vi "Launch Async.vi"(8 "error in (no error)":errorcluster, 10 "Device Ref in":T8 format="%.0x", 11 "RT Data in":T1 {"Channels"."Voltage"."Ref"."Data Reference" format="%.0x"; "Channels"."Current"."Ref"."Data Reference" format="%.0x"; "Channels"."Read Volt"."Ref" format="%.0x"; "Channels"."Mode"."Ref" format="%.0x"}) -> (0 "error out":errorcluster, 2 "Device Ref out":T8 format="%.0x", 3 "RT Data out":T1 {"Channels"."Voltage"."Ref"."Data Reference" format="%.0x"; "Channels"."Current"."Ref"."Data Reference" format="%.0x"; "Channels"."Read Volt"."Ref" format="%.0x"; "Channels"."Mode"."Ref" format="%.0x"})   [LabVIEW 2011, in "Switch-DMM Custom Device.lvlib"]
uses:
  Switch-DMM Custom Device.lvlib
  <vilib>/NI Veristand/Custom Device API/Custom Device Item Ref.ctl
  Controls/RT Data.ctl
  Controls/Channels.ctl
  Controls/Single Channel.ctl
  <vilib>/NI Veristand/Custom Device API/Data Reference.ctl
  Controls/Block Channels.ctl
  <vilib>/NI Veristand/Custom Device API/Block Data Reference.ctl
  Controls/Communication.ctl
  Controls/Async Status.ctl
  Controls/Async State.ctl
  Controls/Async Command.ctl
  Controls/Async Events.ctl
  Controls/Async Data.ctl
  Controls/Hardware.ctl
  <instrlib>/niDMM/nidmm.llb/niDMM Resolution in Digits.ctl
  <vilib>/NI Veristand/Custom Device API/Custom Device API.lvlib
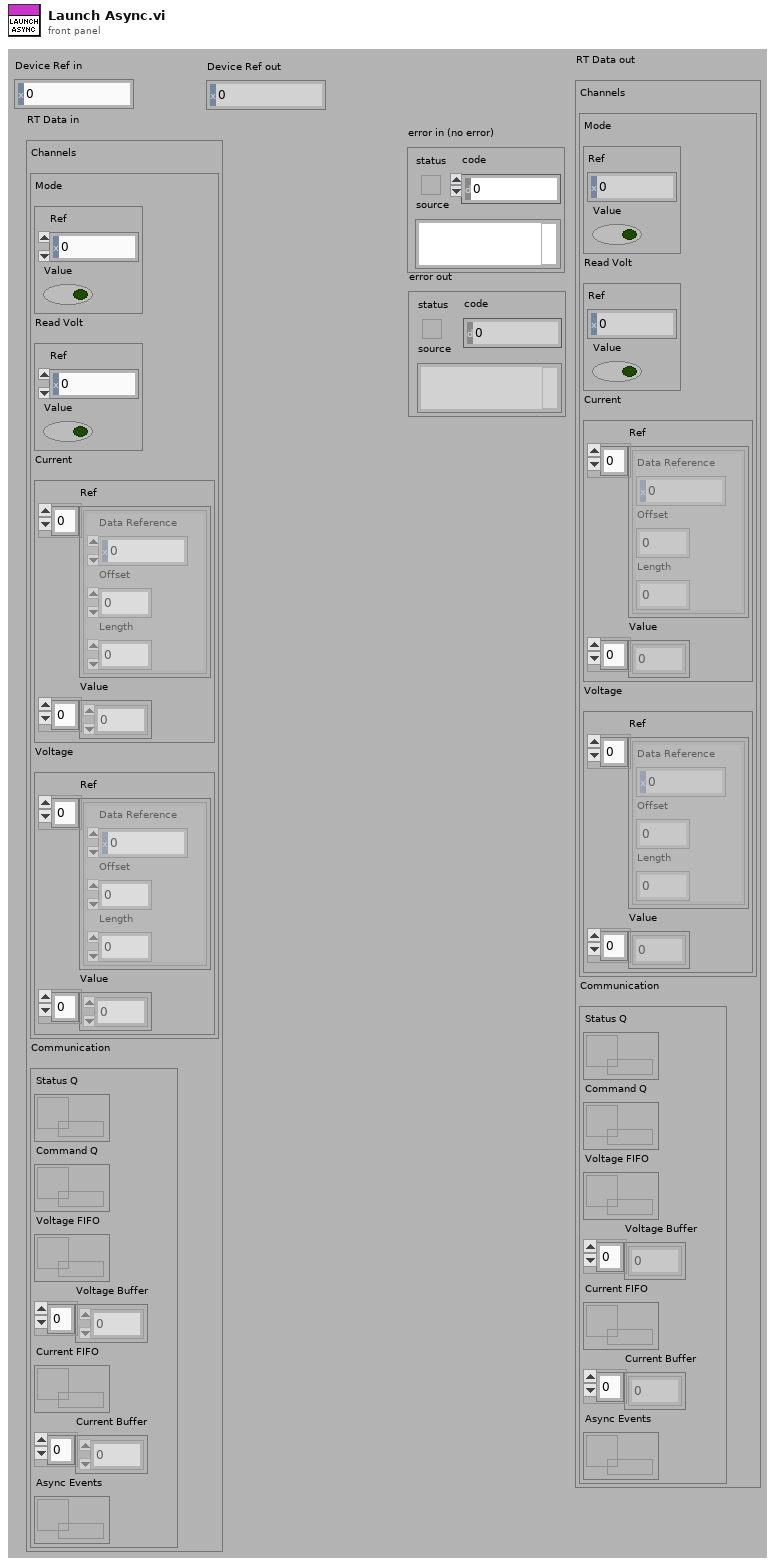
[diagram p1: front panel]
types:
  T1 = typedef "Switch-DMM Custom Device.lvlib/RT Data.ctl" = cluster{"Channels":T2, "Communication":T7}
  T2 = typedef "Switch-DMM Custom Device.lvlib/Channels.ctl" = cluster{"Mode":T3, "Read Volt":T3, "Current":T5, "Voltage":T5}
  T3 = typedef "Switch-DMM Custom Device.lvlib/Single Channel.ctl" = cluster{"Ref":T4, "Value":bool}
  T4 = typedef "Custom Device API.lvlib/Data Reference.ctl" = i32
  T5 = typedef "Switch-DMM Custom Device.lvlib/Block Channels.ctl" = cluster{"Ref":T6[], "Value":dbl[]}
  T6 = typedef "Custom Device API.lvlib/Block Data Reference.ctl" = cluster{"Data Reference":T4, "Offset":i32, "Length":i32}
  T7 = typedef "Switch-DMM Custom Device.lvlib/Communication.ctl" = cluster{"Status Q":refnum<queue>, "Command Q":refnum<queue>, "Voltage FIFO":refnum<k33>, "Voltage Buffer":dbl[], "Current FIFO":refnum<k33>, "Current Buffer":dbl[], "Async Events":refnum<queue>}
  T8 = typedef "Custom Device API.lvlib/Custom Device Item Ref.ctl" = u64
  T9 = typedef "Switch-DMM Custom Device.lvlib/Async Data.ctl" = cluster{"Hardware":T10, "Communication":T7}
  T10 = typedef "Switch-DMM Custom Device.lvlib/Hardware.ctl" = cluster{"Switch Device":refnum<k15>, "DMM Device":refnum<k15>, "DMM -> Switch Trigger":u16, "Switch -> DMM Trigger":u16, "Sample Interval (sec)":dbl, "Current Samples":i32, "Current Limit":dbl, "Current Resolution":T11, "Auto-Read":bool, "Keep Values":bool}
  T11 = typedef "niDMM Resolution in Digits.ctl" = dbl
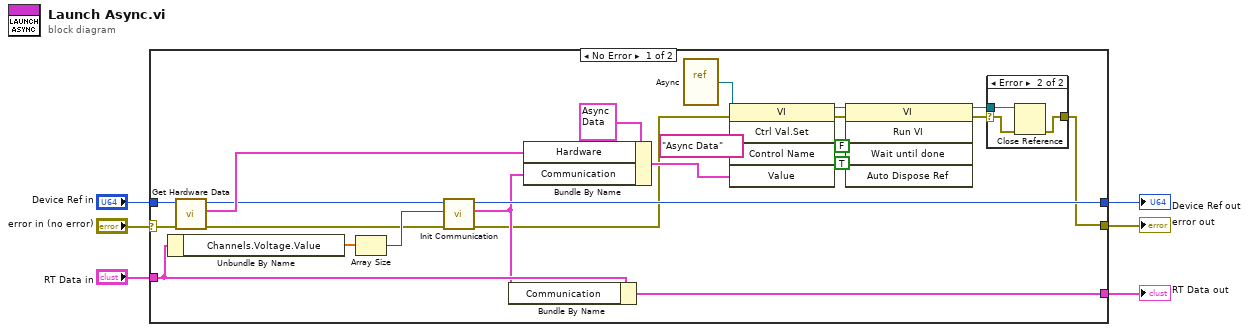
[diagram p0: block diagram]
diagram:
  n1 = case shown="No Error" "error in (no error)" {
    selector: "error in (no error)" -> [w28 w36]
    tunnel: [w9 w36] -> w5
    tunnel: "Device Ref in" -> [w27 w35]
    tunnel: [w25 w35] -> w3
    tunnel: "RT Data in" -> [w22 w34]
    tunnel: [w20 w34] -> w1
    frame No Error {
      n2 = Unbundle By Name(w22) -> ("Channels.Voltage.Value"=w24:dbl[])
      n3 = call "Get Hardware Data.vi"("error in (no error)"=w28, "Device Ref in"=w27) -> ("error out"=w7:errorcluster, "Hardware"=w26:T10, "Item Ref out"=w8:T8)  [unwired: 7 in]
      n4 = Array Size(array=w24) -> (size(s)=w23:i32)
      n5 = call "Init Communication.vi"("error in (no error)"=w7, "Voltage Length"=w23, "Item Ref in"=w8) -> ("error out"=w10:errorcluster, "Communication"=w21:T7, "Item Ref out"=w25:T8)  [unwired: 6 in]
      n6 = Bundle By Name(cluster=w22, "Communication"=w21) -> (w20:T1)
      n7 = Bundle By Name(cluster=T9 {"Hardware"={"Switch Device"="", "DMM Device"="", "DMM -> Switch Trigger"=0, "Switch -> DMM Trigger"=0, "Sample Interval (sec)"=0.0, "Current Samples"=0, "Current Limit"=0.0, "Current Resolution"=0.0, "Auto-Read"=FALSE, "Keep Values"=FALSE}, "Communication"={"Status Q"=refnum, "Command Q"=refnum, "Voltage FIFO"=refnum, "Voltage Buffer"=[], "Current FIFO"=refnum, "Current Buffer"=[], "Async Events"=refnum}} ("Async Data"), "Hardware"=w26, "Communication"=w21) -> (w12:T9)
      n8 = vi-ref "Async.vi"() -> (w13:refnum<vi>)
      n9 = invoke class="VI" method="Ctrl Val.Set"(reference=w13, error in=w10, "Control Name"="Async Data", "Value"=w12) -> (reference out=w19:refnum<vi>, error out=w18:errorcluster)  [unwired: 1 in, 3 out]
      n10 = invoke class="VI" method="Run VI"(reference=w19, error in=w18, "Wait until done"=FALSE ("Wait Until Done"), "Auto Dispose Ref"=TRUE ("Auto Dispose Reference")) -> (reference out=w14:refnum<vi>, error out=w15:errorcluster)  [unwired: 1 in, 3 out]
      n11 = case shown="Error" w15 {
        selector: w15 -> [w30 w32]
        tunnel: w14 -> [_ w33]
        tunnel: [w30 w31] -> w9
        frame No Error {
        }
        frame Error {
          n12 = Close Reference(reference=w33, error in (no error)=w32) -> (error out=w31:errorcluster)
        }
      }
    }
    frame Error {
    }
  }
  "error out" <- w5
  "Device Ref out" <- w3
  "RT Data out" <- w1
